vi "Router - Interelaved Ch - Throughput.vi"() -> ()   [LabVIEW 2016]
uses:
  <vilib>/Utility/error.llb/DialogType.ctl
  <vilib>/Platform/TimedLoop/XDataNode/timing_clust.ctl
  <vilib>/Platform/TimedLoop/XDataNode/nitl_modes.ctl
  <vilib>/Platform/TimedLoop/XDataNode/wakeup.ctl
  <vilib>/pximc/Initialize Reader Session (DBL).vi
  <vilib>/pximc/Connect (DBL).vi
  <vilib>/pximc/Acquire Read Region (DBL).vi
  <vilib>/platform/TimedLoop/XDataNode/XDataNode.xnode
  <vilib>/pximc/nipximc.lvlib
  <resource>/objmgr/pximc.rc
  <vilib>/Platform/TimedLoop/XDataNode/XDNodeRunTimeDep.lvlib
panel:
  out "Throughput S/s":dbl format="%#.2p"
  out "Time has Elapsed":bool
  in  "#Reading Channels Slave 1":i32=4
  in  "Stop Button":bool
  in  "Node 1 Reader Interface":tag="PXI1Slot2" caption="interface"
  in  "Buffer Size":u64=250000 caption="buffer size"
  in  "Connection Timeout (s)":dbl=60.0 caption="timeout in seconds (-1)"
  in  "Node 1 Reader Connection ID":u16=1
  # "Node 1"
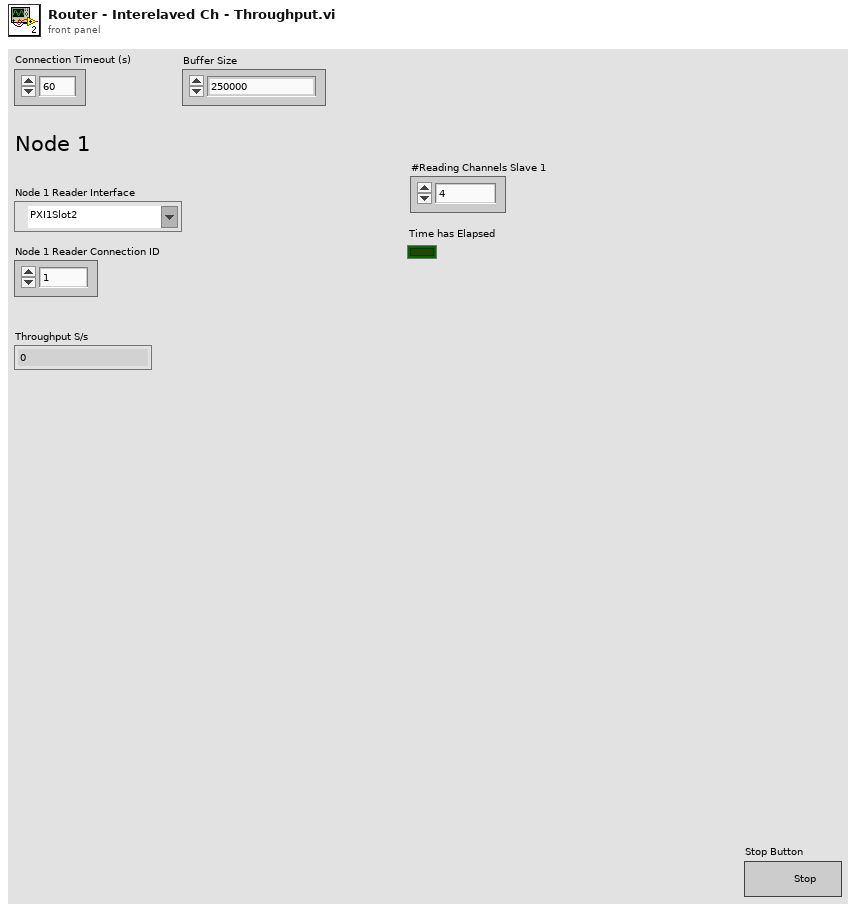
[diagram p1: front panel]
types:
  T1 = typedef "DialogType.ctl" = u16
  T2 = typedef "XDNodeRunTimeDep.lvlib/timing_clust.ctl" = cluster{"Expected End [f-1]":u64, "Actual End [f-1]":u64, "Finished Late? [f-1]":bool, "Expected End [i-1]":u64, "Actual End [i-1]":u64, "Finished Late? [i-1]":bool, "Expected Start [i]":u64, "Actual Start [i]":u64, "Expected Start [f]":u64, "Actual Start [f]":u64, "Source Name":string, "Structure Name":string, "Period":i64, "Deadline":i64, "Offset":i64, "Start":i64, "Priority":i32, "Timeout":i32, "Mode":T3, "Wakeup Reason":T4, "Error":errorcluster, "Source Type":string, "Secondary Source Type":string, "Global End Time":u64, "Global Start Time":u64, "Frame Duration":u64, "Iteration Duration":u64, "Assigned CPU":i32, "I/O Scan Engine Mode":u32}
  T3 = typedef "XDNodeRunTimeDep.lvlib/nitl_modes.ctl" = enum32{"No Change", "Process missed periods, maintain original phase", "Discard missed periods, maintain original phase", "Process missed periods, ignore original phase", "Discard missed periods, ignore original phase"}
  T4 = typedef "XDNodeRunTimeDep.lvlib/wakeup.ctl" = enum32{"Normal", "Aborted", "Asynchronous wakeup", "Timing source error", "Timed loop error", "Timeout"}
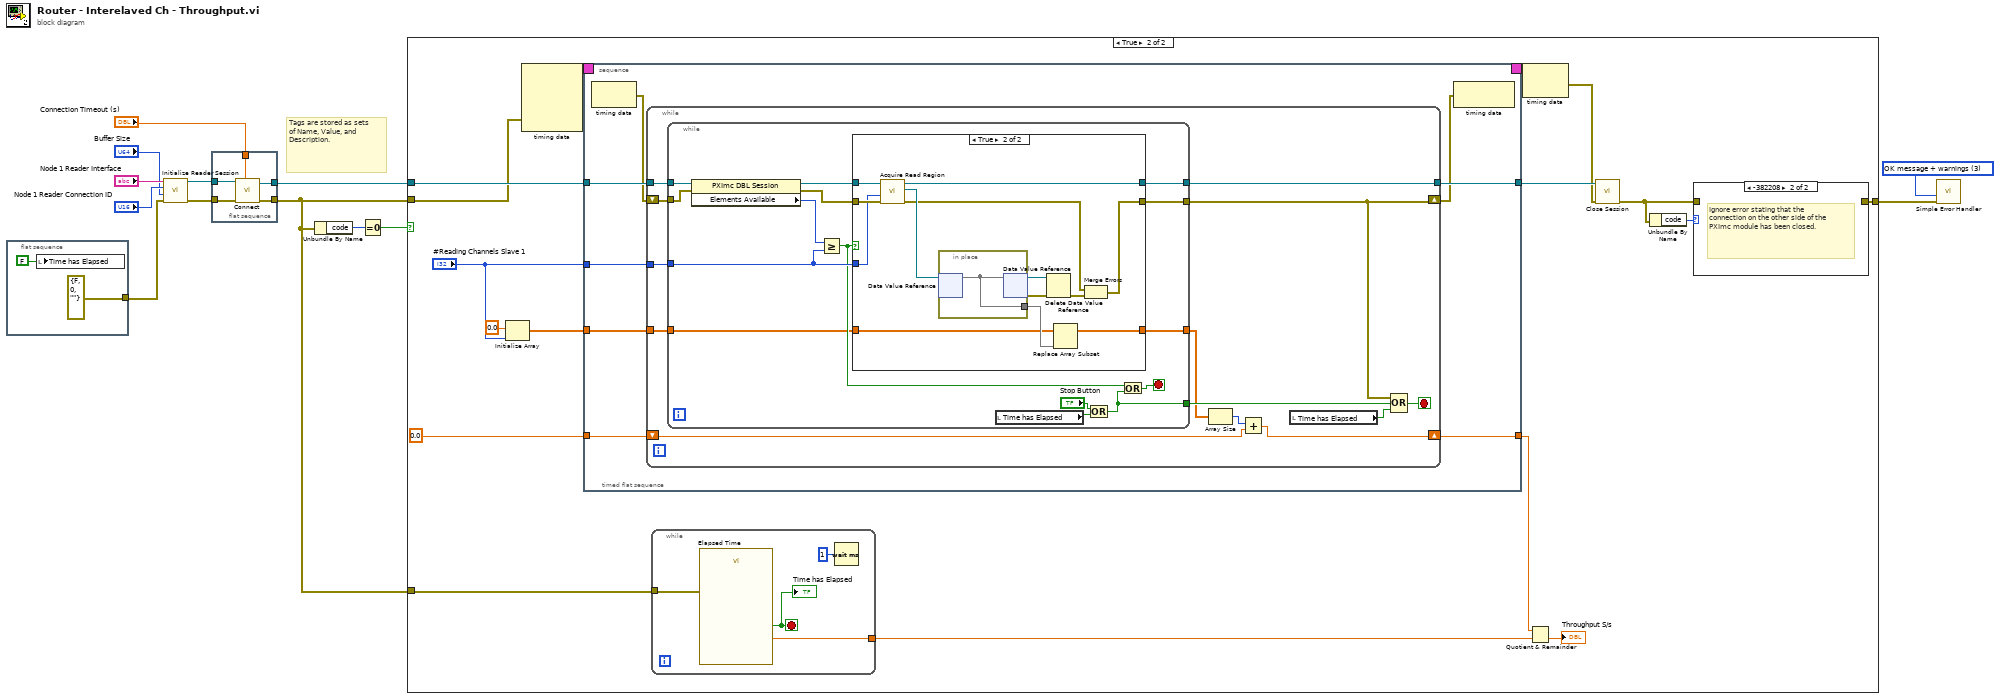
[diagram p0: block diagram]
diagram:
  w8 = T1 3 items=["no dialog", "OK message", "continue or stop message", "OK message + warnings", "continue/stop + warnings"] ("type of dialog (OK msg:1)")
  # "Tags are stored as sets of Name, Value, and Description."
  n1 = flat-sequence {
    tunnel: [errorcluster {"status"=FALSE, "code"=0, "source"=""} ("error constant")] -> w1
    frame #0 {
      n2 = local write "Time has Elapsed"(FALSE ("Stopped?")) -> ()
    }
  }
  n3 = call-poly <vilib>:"Initialize Reader Session.vi"("error in (no error)"=w1, "buffer size"="Buffer Size", "writer's connection id (1)"="Node 1 Reader Connection ID", "interface"="Node 1 Reader Interface") -> ("error out"=w11:errorcluster, "session out"=w12:refnum<k21>)  [unwired: 6 in]
  n4 = flat-sequence {
    tunnel: w12 -> [w20]
    tunnel: w11 -> [w19]
    tunnel: [w18] -> w4
    tunnel: [w17] -> w2
    tunnel: "Connection Timeout (s)" -> [w16]
    frame #0 {
      n5 = call-poly <vilib>:"Connect.vi"("timeout in seconds (-1)"=w16, "error in (no error)"=w19, "session in"=w20) -> ("error out"=w17:errorcluster, "session out"=w18:refnum<k21>)  [unwired: 7 in]
    }
  }
  n6 = Unbundle By Name(w2) -> ("code"=w9:i32)
  n7 = Equal To 0?(x=w9) -> (x = 0?=w3:bool)
  n8 = case shown="True" w3 {
    tunnel: [w21 w36] -> w5
    tunnel: w2 -> [w21 w22]
    tunnel: w4 -> [_ w35]
    tunnel: w2 -> [_ w32]
    frame False {
    }
    frame True {
      n9 = Initialize Array(0.0 ("element"), "#Reading Channels Slave 1") -> (w26:dbl[])
      n10 = node-c288(w22) -> (w25:T2)  [unwired: 3 in]
      n11 = timed-sequence {
        timing: w25 -> [_]
        timing-out: [_] -> w24
        tunnel: w35 -> [w44]
        tunnel: [w43] -> w34
        tunnel: 0.0 ("element") -> [w42]
        tunnel: [w41] -> w31
        tunnel: "#Reading Channels Slave 1" -> [w40]
        tunnel: w26 -> [w39]
        n12 = timed-flat-sequence {
          tunnel: w44 -> [w52]
          tunnel: [w51] -> w43
          tunnel: w42 -> [w50]
          tunnel: [w49] -> w41
          tunnel: w40 -> [w48]
          tunnel: w39 -> [w47]
          n13 = node-c288() -> (w46:errorcluster)  [unwired: 1 in]
          n14 = while {
            tunnel: [w63] -> w51
            shift-right: [w62] -> w45
            shift-left: w46 -> [w61]
            tunnel: w52 -> [w64]
            shift-right: [w58] -> w49
            shift-left: w50 -> [w59]
            tunnel: w48 -> [w54]
            tunnel: w47 -> [w53]
            stop <- w65 stop-if-true
            n15 = while {
              tunnel: w64 -> [w79]
              tunnel: w61 -> [w76]
              tunnel: [w80] -> w62
              tunnel: w54 -> [w73]
              tunnel: [w72] -> w63
              tunnel: [w67] -> w60
              tunnel: [w74] -> w56
              tunnel: w53 -> [w66]
              stop <- w70 stop-if-true
              n16 = property class="PXImc DBL Session"(reference=w79, error in=w76) -> (reference out=w77:refnum<k21>, error out=w75:errorcluster, "Elements Available"=w78:u64)
              n17 = Greater Or Equal?(x=w78, y=w73) -> (x >= y?=w71:bool)
              n18 = case shown="True" w71 {
                tunnel: w75 -> [w83 w95]
                tunnel: [w83 w89] -> w80
                tunnel: w77 -> [w82 w94]
                tunnel: [w81 w86] -> w74
                tunnel: w73 -> [_ w88]
                tunnel: [w82 w87] -> w72
                tunnel: w66 -> [w81 w84]
                frame False {
                }
                frame True {
                  n19 = call-poly <vilib>:"Acquire Read Region.vi"("error in (no error)"=w95, "number of elements"=w88, "session in"=w94) -> ("error out"=w90:errorcluster, "read region reference"=w96:refnum<data-value>, "session out"=w87:refnum<k21>)  [unwired: 5 in, 1 out]
                  n20 = in-place {
                    in-place-border: [w97] -> w85
                    n21 = in-place-dvr #1(w96) -> (w97:dbl[])  [unwired: 1 out]
                    n22 = in-place-dvr #1(w97) -> (w93:refnum<data-value>, w92:errorcluster)
                  }
                  n23 = Delete Data Value Reference(data value reference=w93, error in=w92) -> (error out=w91:errorcluster)  [unwired: 1 out]
                  n24 = Replace Array Subset(array=w84, new element=w85) -> (w86:dbl[])  [unwired: 1 in]
                  n25 = Merge Errors(w90, w91) -> (w89:errorcluster)
                }
              }
              n26 = local read "Time has Elapsed"() -> (w68:bool)
              n27 = Or(x="Stop Button", y=w68) -> (x .or. y?=w67:bool)
              n28 = Or(x=w71, y=w67) -> (x .or. y?=w70:bool)
            }
            n29 = Array Size(array=w56) -> (size(s)=w55:i32)
            n30 = Add(x=w55, y=w59) -> (x+y=w58:dbl)
            n31 = local read "Time has Elapsed"() -> (w57:bool)
            n32 = Compound Arithmetic op=OR(w62, w60, w57) -> (w65:bool)
          }
          n33 = node-c288(w45) -> ()  [unwired: 1 out]
        }
      }
      n34 = while {
        tunnel: w32 -> [w110]
        tunnel: [w109] -> w30
        stop <- w111 stop-if-true
        n35 = call "Elapsed Time"("error in (no error)"=w110) -> ("Elapsed Time (s)"=w109:dbl, "Time has Elapsed"=w111:bool)  [unwired: 11 in, 6 out]
        "Time has Elapsed" <- w111
        n36 = Wait (ms)(milliseconds to wait=u32 1) -> ()  [unwired: 1 out]
      }
      n37 = node-c288(w24) -> (w23:errorcluster)
      n38 = Quotient & Remainder(x=w31, y=w30) -> (floor(x/y)=→"Throughput S/s":dbl)  [unwired: 1 out]
      n39 = call <vilib>:"Close Session.vi"("error in (no error)"=w23, "session in"=w34) -> ("error out"=w37:errorcluster)  [unwired: 9 in]
      n40 = Unbundle By Name(w37) -> ("code"=w38:i32)
      n41 = case shown="-382208" w38 {
        tunnel: w37 -> [w112 _]
        tunnel: [w112 _] -> w36
        frame 0, Default {
        }
        frame -382208 {
          # "Ignore error stating that the connection on the other side of the PXImc module has been closed."
        }
      }
    }
  }
  n42 = call <vilib>:"Simple Error Handler.vi"("type of dialog (OK msg:1)"=w8, "error in (no error)"=w5) -> ()  [unwired: 3 in, 5 out]
